vi "Gen_Sin_w_ShotNoise.vi"(2 "[IN] Ampl. Shot Noise, 0...1":dbl=0.2, 3 "[IN] Amplitude":dbl=1.0, 4 "[IN] X value":dbl) -> (0 "[OUT] Value":dbl)   [LabVIEW 2022 SP3]
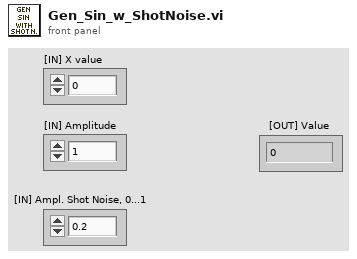
[diagram p1: front panel]
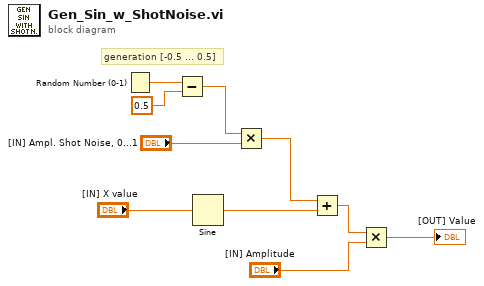
[diagram p0: block diagram]
diagram:
  # "generation [-0.5 ... 0.5]"
  n1 = Random Number (0-1)() -> (number: 0 to 1=w9:dbl)
  n2 = Subtract(x=w9, y=0.5) -> (x-y=w4:dbl)
  n3 = Sine(x="[IN] X value") -> (sin(x)=w7:dbl)
  n4 = Multiply(x=w4, y="[IN] Ampl. Shot Noise, 0...1") -> (x*y=w2:dbl)
  n5 = Add(x=w2, y=w7) -> (x+y=w6:dbl)
  n6 = Multiply(x=w6, y="[IN] Amplitude") -> (x*y=→"[OUT] Value":dbl)
